vi "GetStatusMDrive.vi"(0 "Channel Properties":T1={"Channel Name"="", "Vel. Default"=5.0, "Acc. Default"=5.0, "Vel. Max"=5.0, "Vel. Min"=5.0, "Acc. Max"=5.0, "Acc. Min"=5.0, "Pulses/unit"=0.0, "Address"=0, "Pulse Offset"=0, "Pos Tolerance"=0.0, "Pulses/rev"=0.0, "Backlash/Eng units"=0.0, "Current Pos"=0.0, "Ch Status"=enum."Active", "Port Name"="", "Axis Transform mode"="", "Metadata Ch Name"="", "Type"=""} {"Current Pos" format="%.2f"; "Backlash/Eng units" format="%.2f"; "Pulses/rev" format="%.2f"; "Pos Tolerance" format="%.2f"; "Pulses/unit" format="%.2f"; "Acc. Min" format="%.2f"; "Acc. Max" format="%.2f"; "Vel. Min" format="%.2f"; "Vel. Max" format="%.2f"; "Acc. Default" format="%.2f"; "Vel. Default" format="%.2f"}, 2 "Limit switch valid?":bool, 3 "Stop on Trigger 3?":bool) -> (5 "Ready":bool, 6 "OK":bool, 7 "Position in Move":dbl format="%.2f", 8 "Error string":string)   [LabVIEW 2011]
uses:
  ~subVIs/DriveProperties.ctl
  ~subVIs/GenericDriveCommand.ctl
  MDriveDriveCommand.ctl
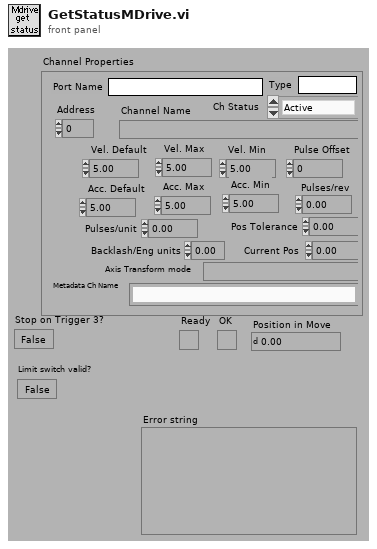
[diagram p1: front panel]
types:
  T1 = typedef "DriveProperties.ctl" = cluster{"Channel Name":string, "Vel. Default":dbl, "Acc. Default":dbl, "Vel. Max":dbl, "Vel. Min":dbl, "Acc. Max":dbl, "Acc. Min":dbl, "Pulses/unit":dbl, "Address":u8, "Pulse Offset":i32, "Pos Tolerance":dbl, "Pulses/rev":dbl, "Backlash/Eng units":dbl, "Current Pos":dbl, "Ch Status":enum16{"Active", "Offline", "Simulate"}, "Port Name":string, "Axis Transform mode":string, "Metadata Ch Name":string, "Type":string}
  T2 = typedef "GenericDriveCommand.ctl" = string
  T3 = typedef "MDriveDriveCommand.ctl" = string
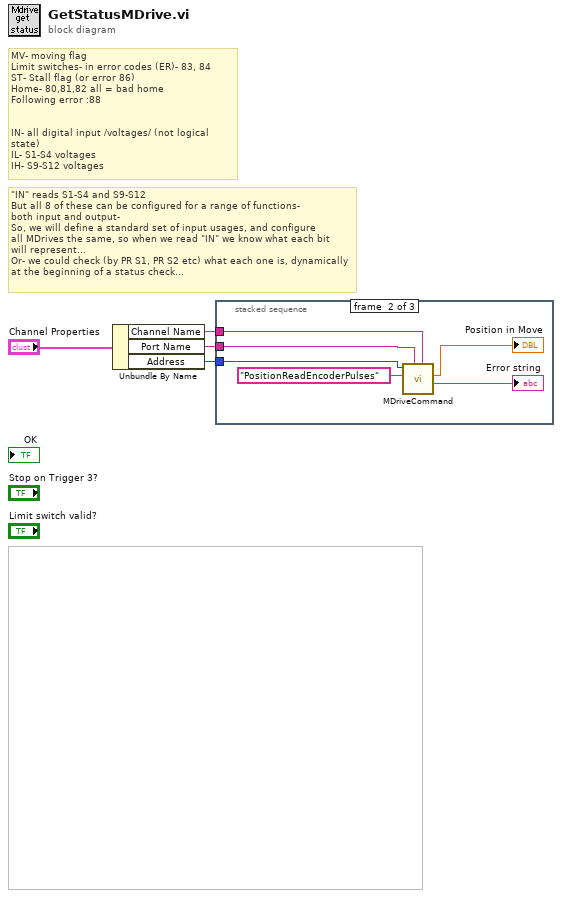
[diagram p0: block diagram]
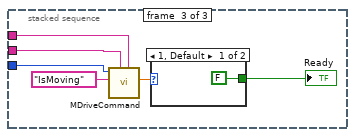
[diagram p3: hidden frame]
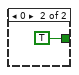
[diagram p4: hidden frame]
diagram:
  # "\"IN\" reads S1-S4 and S9-S12\nBut all 8 of these can be configured for a range of functions-\nboth input and output-\nSo, we will define a standard set of input usages, and configure\nall MDrives the same, so when we read \"IN\" we know what each bit \nwill represent...\nOr- we could check (by PR S1, PR S2 etc) what each one is, dynamically\nat the beginning of a status check..."
  # "MV- moving flag\nLimit switches- in error codes (ER)- 83, 84\nST- Stall flag (or error 86)\nHome- 80,81,82 all = bad home\nFollowing error :88\n\n\nIN- all digital input /voltages/ (not logical state)\nIL- S1-S4 voltages\nIH- S9-S12 voltages"
  n1 = Unbundle By Name("Channel Properties") -> ("Channel Name"=w1:string, "Port Name"=w3:string, "Address"=w2:u8)
  n2 = stacked-sequence {
    tunnel: w3 -> [_ w10 w16]
    tunnel: w2 -> [_ w9 w15]
    tunnel: w1 -> [_ w8 w14]
    frame #0 {
    }
    frame #1 {
      n3 = call "MDriveCommand.vi"("Channel Name"=w8, "Port Name"=w10, "MDriveCommand"=T2 "PositionReadEncoderPulses" ("GenericDriveCommand"), "Address"=w9) -> ("Error Description"=→"Error string":string, "Numeric Reply"=→"Position in Move":dbl)  [unwired: 2 in, 3 out]
    }
    frame #2 {
      n4 = call "MDriveCommand.vi"("Channel Name"=w14, "Port Name"=w16, "MDriveCommand"=T3 "IsMoving" ("DriveCommand"), "Address"=w15) -> ("Numeric Reply"=w12:dbl)  [unwired: 2 in, 4 out]
      n5 = case shown="1, Default" w12 {
        tunnel: [FALSE ("Ready") TRUE ("Ready")] -> w11
        frame 1, Default {
        }
        frame 0 {
        }
      }
      "Ready" <- w11
    }
  }
